vi "Projecdt ini info.vi"() -> ()   [LabVIEW 2010]
uses:
  GUI/Job setup/Job and site cluster.ctl
  emi cndiates/List of all contrys(combo box).ctl
  GUI/Job setup/Tool registration ID.ctl
  GUI/Job setup/Operators display clustor.ctl
panel:
  out "Project information":T5
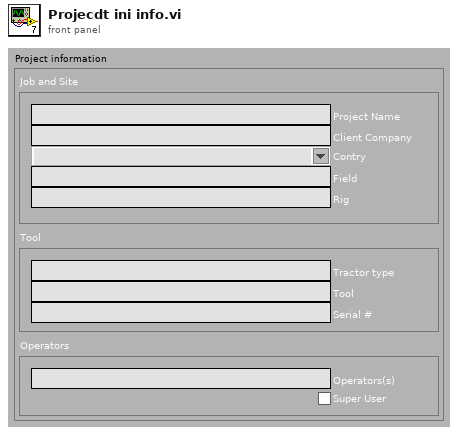
[diagram p1: front panel]
types:
  T1 = typedef "Job and site cluster.ctl" = cluster{"Project Name":string, "Client Company":string, "Field":string, "Rig":string, "Contry":T2}
  T2 = typedef "List of all contrys(combo box).ctl" = string
  T3 = typedef "Tool registration ID.ctl" = cluster{"Tractor type":string, "Tool":string, "Serial #":string}
  T4 = typedef "Operators display clustor.ctl" = cluster{"Operators(s)":string, "Super User":bool}
  T5 = cluster{"Job and Site":T1, "Tool":T3, "Operators":T4}
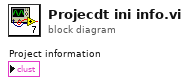
[diagram p0: block diagram]
diagram:
